vi "Write Prepend Minion ID.vi"(8 "error in (no error)":errorcluster, 10 "Prepend Minion ID":bool, 11 "SystemLink configuration in":refnum<class "SystemLink configuration.lvclass">) -> (0 "error out":errorcluster, 3 "SystemLink configuration out":refnum<class "SystemLink configuration.lvclass">)   [LabVIEW 2015, in "SystemLink configuration.lvclass"]
uses:
  SystemLink configuration.lvclass
  SystemLink configuration.lvclass/SystemLink configuration.ctl
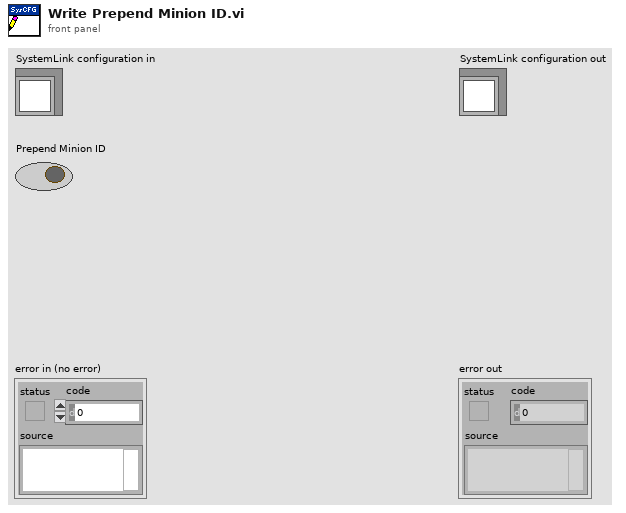
[diagram p1: front panel]
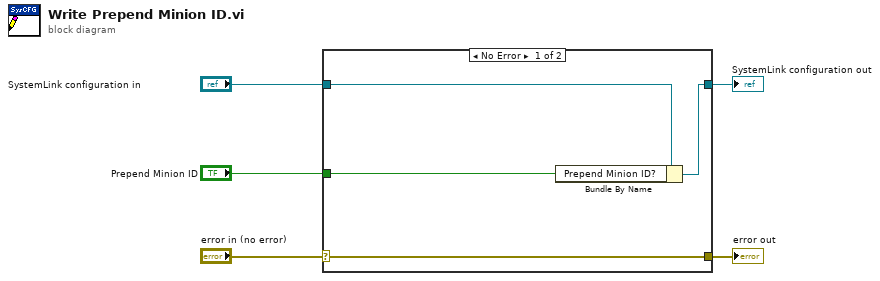
[diagram p0: block diagram]
diagram:
  n1 = case shown="No Error" "error in (no error)" {
    selector: "error in (no error)" -> [w9 w10]
    tunnel: [w9 w10] -> w4
    tunnel: [w7 w11] -> w2
    tunnel: "SystemLink configuration in" -> [w8 w11]
    tunnel: "Prepend Minion ID" -> [w6 _]
    frame No Error {
      n2 = Bundle By Name(cluster=w8, "Prepend Minion ID?"=w6) -> (w7:refnum<class "SystemLink configuration.lvclass">)
    }
    frame Error {
    }
  }
  "error out" <- w4
  "SystemLink configuration out" <- w2
